vi "Set Fault Configuration.vi"(6 "error in (no error)":errorcluster, 8 "fault configuration":T1={"code"=0, "level or level before threshold"=0, "occurrence threshold"=0, "time window in seconds"=0, "level after threshold"=1} {"level after threshold" items=["Ignore"=-1, "Minor"=0, "Major"=1]; "level or level before threshold" items=["Ignore"=-1, "Minor"=0, "Major"=1]}, 9 "target address (localhost)":string="localhost") -> (0 "error out":errorcluster)   [LabVIEW 2017, in "Config Faults.lvlib"]
doc: "Applies a custom fault configuration for a configurable fault."
uses:
  <vilib>/NIScanEngine/ConfigurableFaults/Config Faults.lvlib
  <vilib>/NIScanEngine/ConfigurableFaults/Fault Desc Control.ctl
  <resource>/objmgr/ni.var.rc
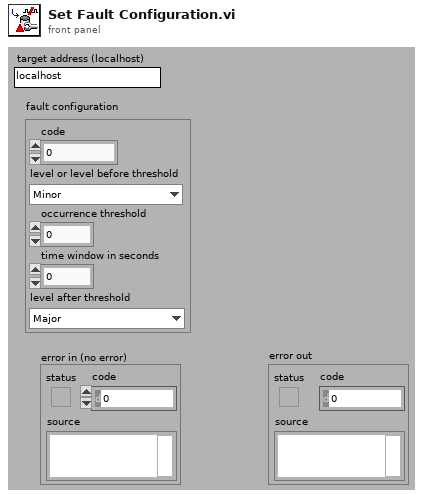
[diagram p1: front panel]
types:
  T1 = typedef "Config Faults.lvlib/Fault Desc Control.ctl" = cluster{"code":i32, "level or level before threshold":i32, "occurrence threshold":u32, "time window in seconds":u32, "level after threshold":i32}
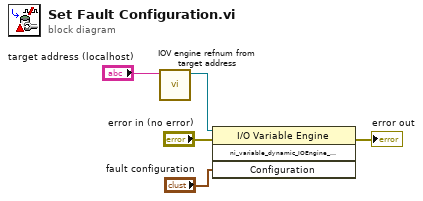
[diagram p0: block diagram]
diagram:
  n1 = call <vilib>:"IOV engine refnum from target address.vi"("target address"="target address (localhost)") -> ("reference out"=w3:refnum<k21>)  [unwired: 10 in]
  n2 = invoke class="I/O Variable Engine" method="ni_variable_dynamic_IOEngine_AddFaultConfig"(reference=w3, error in="error in (no error)", "Configuration"="fault configuration") -> (error out=→"error out":errorcluster)  [unwired: 1 in, 3 out]
